vi "String Indicator.vi"(10 "String Indicator":string, 11 "Dev Panel in":refnum<class "Dev Panel.lvclass">) -> (3 "Dev Panel out":refnum<class "Dev Panel.lvclass">)   [LabVIEW 2021, in "Dev Panel.lvclass"]
uses:
  Dev Panel.lvclass
  Dev Panel.lvclass/Dev Panel.ctl
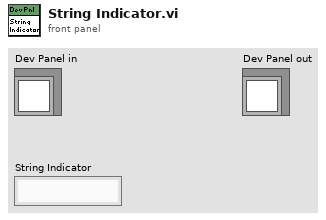
[diagram p1: front panel]
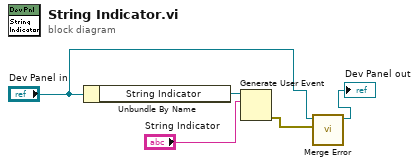
[diagram p0: block diagram]
diagram:
  n1 = Unbundle By Name("Dev Panel in") -> ("String Indicator"=w5:refnum<user-event>)
  n2 = Generate User Event(user event=w5, event data cluster="String Indicator") -> (error out=w3:errorcluster)  [unwired: 2 in, 1 out]
  n3 = call-dynamic "Merge Error.vi"("Error"=w3, "Set Error in"="Dev Panel in") -> ("Set Error out"=→"Dev Panel out":refnum<class "Dev Panel.lvclass">)  [unwired: 9 in]
